vi "Open Database Configuration.vi"(8 "Error In":errorcluster) -> (0 "Error Out":errorcluster, 2 "Database Connection":T1={"Data Source Name"="HANSPH_LAPTOP\\SQLEXPRESS", "Database Name"="MEASUREMENTS", "User Name"="sa", "Password"="Ullabella72"})   [LabVIEW 2018]
uses:
  <vilib>/Utility/config.llb/Read Key (String).vi
  <vilib>/Utility/config.llb/NI_LVConfig.lvlib
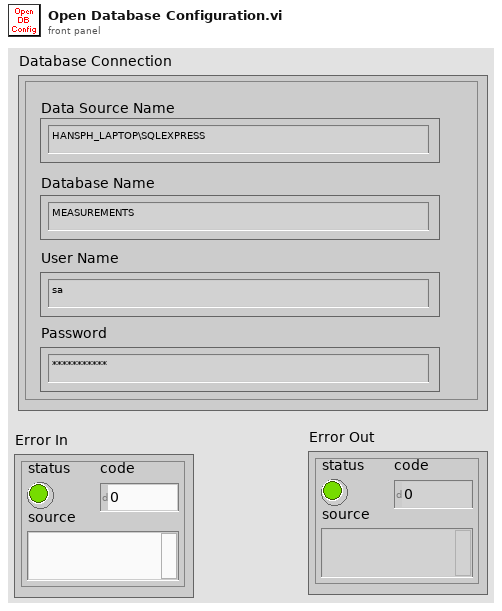
[diagram p1: front panel]
types:
  T1 = cluster{"Data Source Name":string, "Database Name":string, "User Name":string, "Password":string}
  T2 = typedef "NI_LVConfig.lvlib/Config Data RefNum.ctl" = refnum<k1>
  T3 = cluster{"value":string, "value":string, "value":string, "value":string}
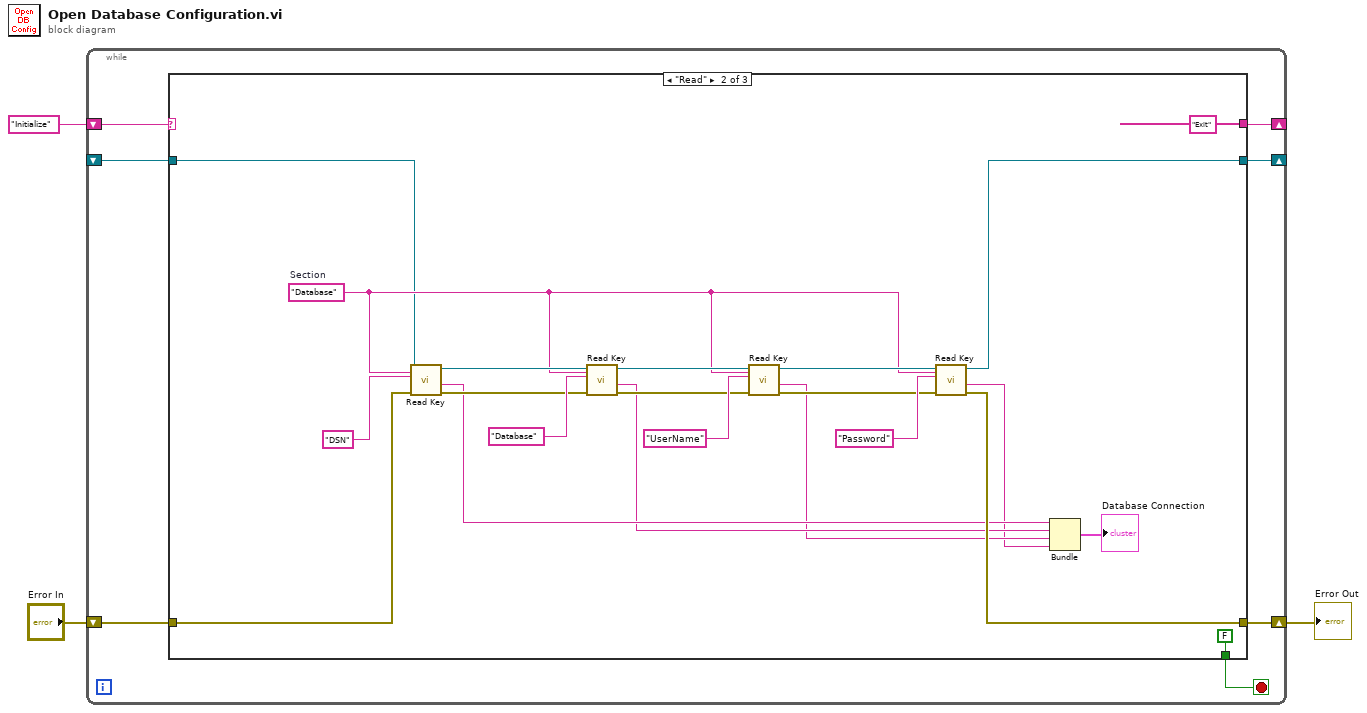
[diagram p0: block diagram]
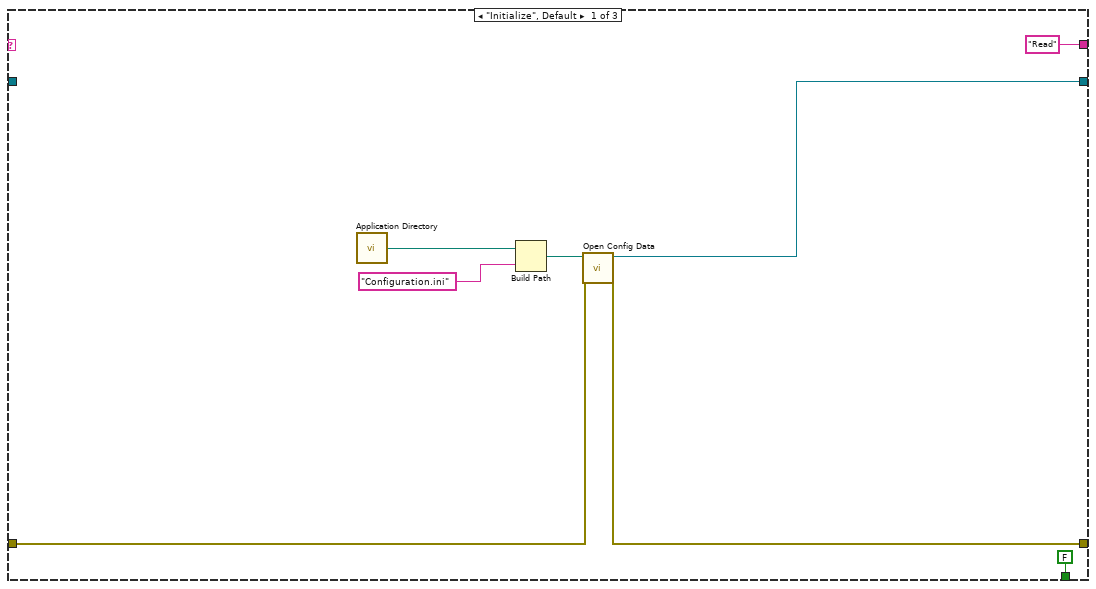
[diagram p2: hidden frame]
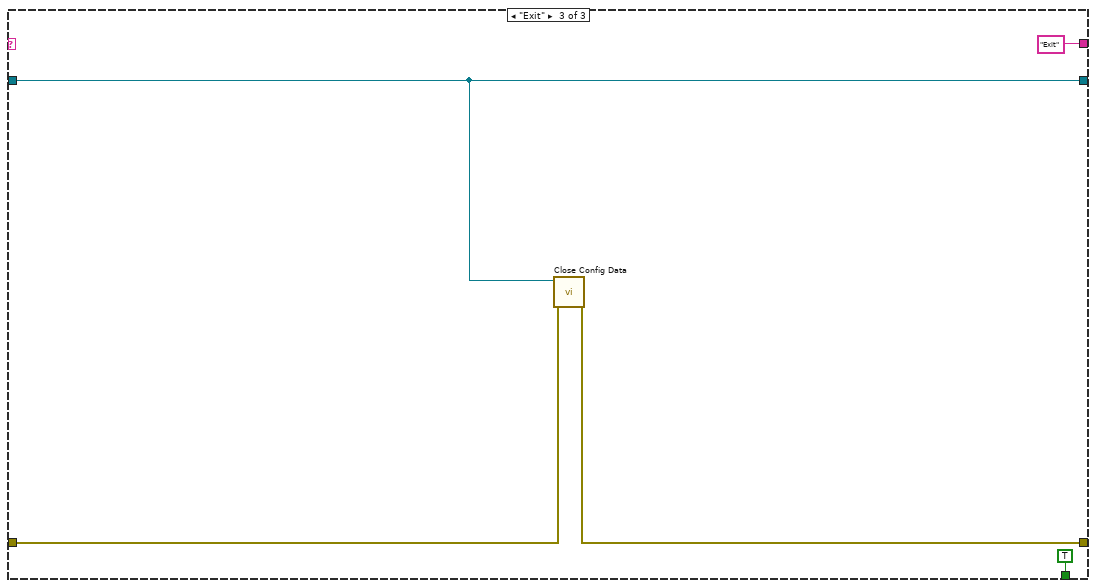
[diagram p3: hidden frame]
diagram:
  n1 = while {
    shift-right: [w6] -> _
    shift-left: "Initialize" ("key") -> [w10]
    shift-right: [w7] -> _
    shift-left: _ -> [w9]
    shift-right: [w4] -> w1
    shift-left: "Error In" -> [w8]
    stop <- w5 stop-if-true
    n2 = case shown="\"Read\"" w10 {
      tunnel: w9 -> [_ w25 w43]
      tunnel: w8 -> [w12 w27 w42]
      tunnel: [w13 w24 w43] -> w7
      tunnel: ["Read" ("key") "Exit" ("key") "Exit" ("key")] -> w6
      tunnel: [FALSE FALSE TRUE] -> w5
      tunnel: [w11 w26 w41] -> w4
      frame "Initialize", Default {
        n3 = call <vilib>:"Application Directory.vi"() -> ("Application Directory"=w16:path)
        n4 = Build Path(base path=w16, name or relative path="Configuration.ini") -> (appended path=w14:path)
        n5 = call <vilib>:"Open Config Data.vi"("error in (no error)"=w12, "configuration file path"=w14) -> ("error out"=w11:errorcluster, "refnum"=w13:T2)  [unwired: 7 in, 1 out]
      }
      frame "Read" {
        w28 = "Database"  # Section
        n6 = call-poly <vilib>:"Read Key.vi"("section"=w28, "error in (no error)"=w27, "key"="DSN", "refnum"=w25) -> ("error out"=w37:errorcluster, "value"=w23:string, "refnum out"=w36:T2)  [unwired: 4 in, 1 out]
        n7 = call-poly <vilib>:"Read Key.vi"("section"=w28, "error in (no error)"=w37, "key"="Database", "refnum"=w36) -> ("error out"=w31:errorcluster, "value"=w22:string, "refnum out"=w32:T2)  [unwired: 4 in, 1 out]
        n8 = call-poly <vilib>:"Read Key.vi"("section"=w28, "error in (no error)"=w31, "key"="UserName", "refnum"=w32) -> ("error out"=w29:errorcluster, "value"=w21:string, "refnum out"=w30:T2)  [unwired: 4 in, 1 out]
        n9 = call-poly <vilib>:"Read Key.vi"("section"=w28, "error in (no error)"=w29, "key"="Password", "refnum"=w30) -> ("error out"=w26:errorcluster, "value"=w20:string, "refnum out"=w24:T2)  [unwired: 4 in, 1 out]
        n10 = Bundle("value"=w23, "value"=w22, "value"=w21, "value"=w20) -> (→"Database Connection":T3)  [unwired: 1 in]
      }
      frame "Exit" {
        n11 = call <vilib>:"Close Config Data.vi"("error in (no error)"=w42, "refnum"=w43) -> ("error out"=w41:errorcluster)  [unwired: 8 in, 1 out]
      }
    }
  }
  "Error Out" <- w1
